vi "Close.vi"(8 "error in (no error)":errorcluster, 11 "TIFF Reader in":refnum<class "TIFF Reader.lvclass">) -> (0 "error out":errorcluster, 3 "path":path)   [LabVIEW 2020, in "LV Tiff.lvlib" / "TIFF Reader.lvclass"]
uses:
  TIFF Reader.lvclass
  TIFF Reader.lvclass/TIFF Reader.ctl
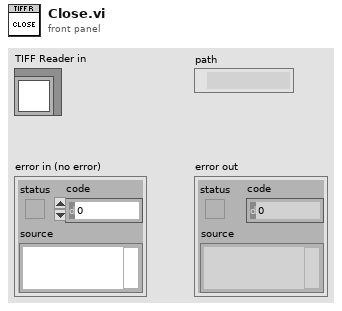
[diagram p1: front panel]
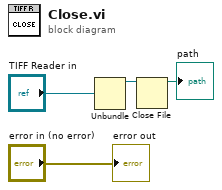
[diagram p0: block diagram]
diagram:
  n1 = Unbundle("TIFF Reader in") -> (w2:refnum<file>)  [unwired: 3 out]
  n2 = Close File(refnum=w2) -> (path=→"path":path)  [unwired: 1 in, 1 out]
  "error out" <- "error in (no error)"
